vi "Restrict X Range.vi"   [LabVIEW 2016, in "xy_utilities.lvlib"]
doc: "Removes data points that fall outside of the range defined by <b>X Min</b> and <b>X Max</b>\n\nWire data to the data input to determine the polymorphic instance to use or manually select the instance."
uses:
  xy_utilities.lvlib
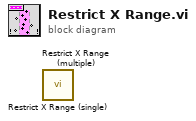
[diagram p0: block diagram]
diagram:
  n1 = call "Restrict X Range (single).vi"() -> ()  [unwired: 10 in, 2 out]
  n2 = call "Restrict X Range (multiple).vi"() -> ()  [unwired: 10 in, 2 out]
